vi "svx_DAQ_ConfigureTask.vi"(0 "Task In":T1, 5 "Display State In":T3={"Channel Info Array"=[], "Timing Mode"=enum."Time", "Timing Control 1"=25600.0, "Timing Control 2"=2560.0, "Timing Control 3"=16, "Timing Indicator 1"=0.1, "Reference Visible?"=FALSE, "Reference Type"=enum."<none>", "Tachometer Channel"="", "Tach Pulses Per Rev"=1, "Tach Direction"=enum."CW", "Tach Slope"=enum."Rising", "Tach Threshold"=0.0, "Trigger Channel"="", "Trigger Level"=20.0, "Pretrigger Samples"=1, "Trigger Slope"=enum."Falling", "Trigger Hysteresis"=0.0, "Logging Visible?"=FALSE, "Enable Logging"=FALSE, "Logfile Path"=path "c:/test.tdms"} caption="State" {"Timing Control 2" format="%#_6f"; "Channel Info Array"."Max" min=0.0 format="± %^#_4g"; "Channel Info Array"."Channel Type" items=["Voltage (V)"=0, "Charge (C)"=9, "-"=99, "SPL (Pa)"=3, "Force (lbf)"=6, "Force (N)"=1, "Acceleration (g) - IEPE"=2, "Acceleration (g) - Charge"=12, "Acceleration (g) - 4 wire DC Voltage"=22, "Velocity (in/s)"=7, "Velocity (mm/s)"=8, "Prox Probe (mil)"=4, "Prox Probe (mm)"=5]}, 9 "cluster":T2, 11 "error in":errorcluster) -> (4 "task out":refnum<k21>, 6 "Display State Out":T3={"Channel Info Array"=[], "Timing Mode"=enum."Time", "Timing Control 1"=25600.0, "Timing Control 2"=2560.0, "Timing Control 3"=16, "Timing Indicator 1"=0.1, "Reference Visible?"=FALSE, "Reference Type"=enum."<none>", "Tachometer Channel"="", "Tach Pulses Per Rev"=1, "Tach Direction"=enum."CW", "Tach Slope"=enum."Rising", "Tach Threshold"=0.0, "Trigger Channel"="", "Trigger Level"=20.0, "Pretrigger Samples"=1, "Trigger Slope"=enum."Falling", "Trigger Hysteresis"=0.0, "Logging Visible?"=FALSE, "Enable Logging"=FALSE, "Logfile Path"=path "c:/test.tdms"} caption="State" {"Timing Control 2" format="%#_6f"; "Channel Info Array"."Max" min=0.0 format="± %^#_4g"; "Channel Info Array"."Channel Type" items=["Voltage (V)"=0, "Charge (C)"=9, "-"=99, "SPL (Pa)"=3, "Force (lbf)"=6, "Force (N)"=1, "Acceleration (g) - IEPE"=2, "Acceleration (g) - Charge"=12, "Acceleration (g) - 4 wire DC Voltage"=22, "Velocity (in/s)"=7, "Velocity (mm/s)"=8, "Prox Probe (mil)"=4, "Prox Probe (mm)"=5]}, 10 "cluster":T2, 15 "error out":errorcluster)   [LabVIEW 2017, in "SVX NI-DAQmx AI Configuration XControl.xctl"]
uses:
  <vilib>/addons/Sound and Vibration/svt_DAQmx/Configuration XControl/SVX NI-DAQmx AI Configuration XControl.xctl
  <vilib>/addons/Sound and Vibration/svt_DAQmx/Configuration XControl/SubVIs/svx_DAQ_State.ctl
  <vilib>/addons/Sound and Vibration/svt_DAQmx/Configuration XControl/Controls/svx_DAQ_ChannelInfo.ctl
  <vilib>/addons/Sound and Vibration/svt_DAQmx/Configuration XControl/Controls/svx_DAQ_ChannelType.ctl
  <vilib>/addons/Sound and Vibration/svt_DAQmx/Configuration XControl/Controls/svx_DAQ_Coupling.ctl
  <vilib>/addons/Sound and Vibration/svt_DAQmx/Configuration XControl/Controls/svx_DAQ_Excitation.ctl
  <vilib>/addons/Sound and Vibration/svt_DAQmx/Configuration XControl/Controls/svx_DAQ_TimingType.ctl
  <vilib>/addons/Sound and Vibration/svt_DAQmx/Configuration XControl/Controls/svx_DAQ_ReferenceType.ctl
  <vilib>/addons/Sound and Vibration/svt_DAQmx/Configuration XControl/Controls/svx_DAQ_RotationDirection.ctl
  <vilib>/addons/Sound and Vibration/svt_DAQmx/Configuration XControl/Controls/svx_DAQ_Tach_Slope.ctl
  <vilib>/addons/Sound and Vibration/svt_DAQmx/Configuration XControl/Controls/svx_DAQ_Trigger_Slope.ctl
  <vilib>/addons/Sound and Vibration/svt_DAQmx/Configuration XControl/Controls/svx_DAQ_ControlRefs.ctl
  <vilib>/addons/Sound and Vibration/svt_DAQmx/Configuration XControl/SubVIs/svx_DAQ_Data.ctl
  <resource>/objmgr/daqmx.rc
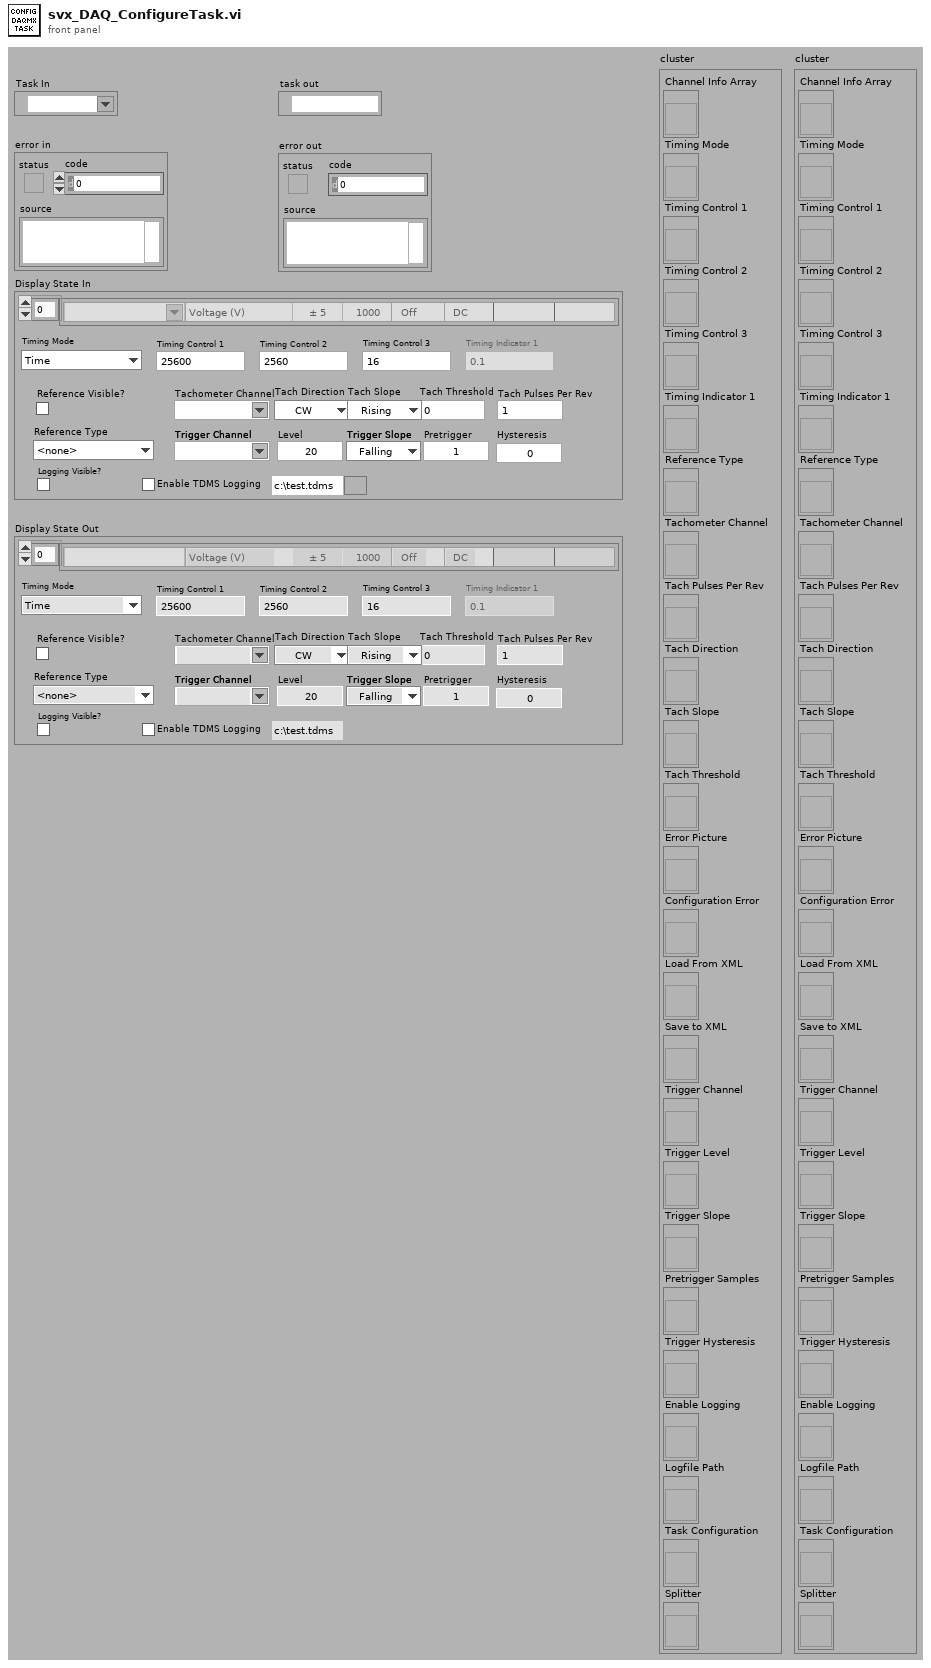
[diagram p1: front panel]
types:
  T1 = typedef "SVX NI-DAQmx AI Configuration XControl.xctl/svx_DAQ_Data.ctl" = refnum<k21>
  T2 = typedef "SVX NI-DAQmx AI Configuration XControl.xctl/svx_DAQ_ControlRefs.ctl" = cluster{"Channel Info Array":refnum<vi>, "Timing Mode":refnum<vi>, "Timing Control 1":refnum<vi>, "Timing Control 2":refnum<vi>, "Timing Control 3":refnum<vi>, "Timing Indicator 1":refnum<vi>, "Reference Type":refnum<vi>, "Tachometer Channel":refnum<vi>, "Tach Pulses Per Rev":refnum<vi>, "Tach Direction":refnum<vi>, "Tach Slope":refnum<vi>, "Tach Threshold":refnum<vi>, "Error Picture":refnum<vi>, "Configuration Error":refnum<vi>, "Load From XML":refnum<vi>, "Save to XML":refnum<vi>, "Trigger Channel":refnum<vi>, "Trigger Level":refnum<vi>, "Trigger Slope":refnum<vi>, "Pretrigger Samples":refnum<vi>, "Trigger Hysteresis":refnum<vi>, "Enable Logging":refnum<vi>, "Logfile Path":refnum<vi>, "Task Configuration":refnum<vi>, "Splitter":refnum<vi>}
  T3 = typedef "SVX NI-DAQmx AI Configuration XControl.xctl/svx_DAQ_State.ctl" = cluster{"Channel Info Array":T4[], "Timing Mode":T8, "Timing Control 1":dbl, "Timing Control 2":dbl, "Timing Control 3":i32, "Timing Indicator 1":dbl, "Reference Visible?":bool, "Reference Type":T9, "Tachometer Channel":string, "Tach Pulses Per Rev":i32, "Tach Direction":T10, "Tach Slope":T11, "Tach Threshold":dbl, "Trigger Channel":string, "Trigger Level":dbl, "Pretrigger Samples":i32, "Trigger Slope":T12, "Trigger Hysteresis":dbl, "Logging Visible?":bool, "Enable Logging":bool, "Logfile Path":path}
  T4 = typedef "SVX NI-DAQmx AI Configuration XControl.xctl/svx_DAQ_ChannelInfo.ctl" = cluster{"Initialized?":bool, "DAQmx Channel":tag, "Channel Type":T5, "Max":dbl, "Sensitivity":dbl, "Excitation":bool, "Coupling":T6, "Location":string, "Orientation":string, "excitation":T7}
  T5 = typedef "SVX NI-DAQmx AI Configuration XControl.xctl/svx_DAQ_ChannelType.ctl" = u16
  T6 = typedef "SVX NI-DAQmx AI Configuration XControl.xctl/svx_DAQ_Coupling.ctl" = enum16{"AC", "DC"}
  T7 = typedef "svx_DAQ_Excitation.ctl" = enum16{"Off", "Min", "Max"}
  T8 = typedef "SVX NI-DAQmx AI Configuration XControl.xctl/svx_DAQ_TimingType.ctl" = enum16{"Time", "Frequency", "Order"}
  T9 = typedef "SVX NI-DAQmx AI Configuration XControl.xctl/svx_DAQ_ReferenceType.ctl" = enum16{"<none>", "Analog Tachometer", "Analog SW Trigger"}
  T10 = typedef "SVX NI-DAQmx AI Configuration XControl.xctl/svx_DAQ_RotationDirection.ctl" = enum16{"CW", "CCW"}
  T11 = typedef "SVX NI-DAQmx AI Configuration XControl.xctl/svx_DAQ_Tach_Slope.ctl" = enum16{"Rising", "Falling"}
  T12 = typedef "SVX NI-DAQmx AI Configuration XControl.xctl/svx_DAQ_Trigger_Slope.ctl" = enum16{"Falling", "Rising"}
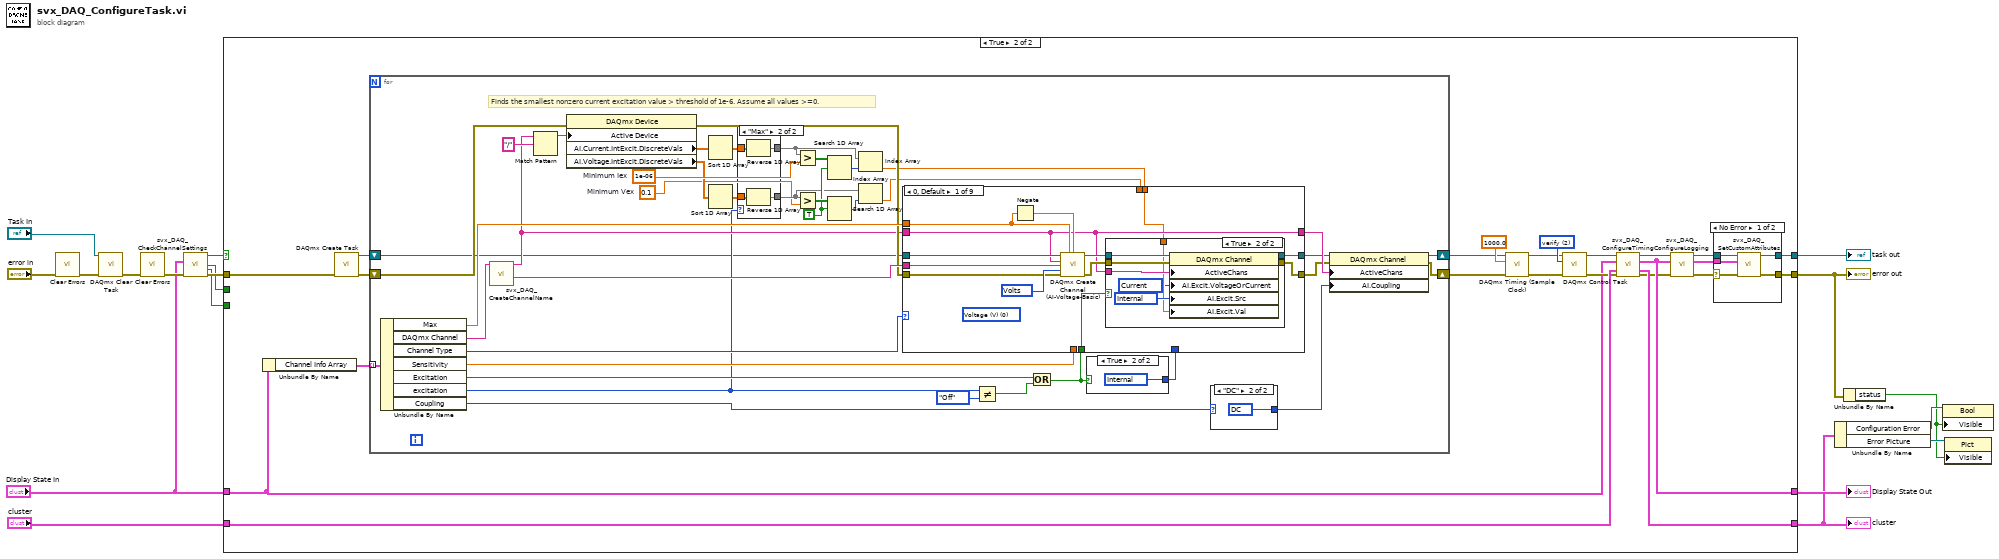
[diagram p0: block diagram]
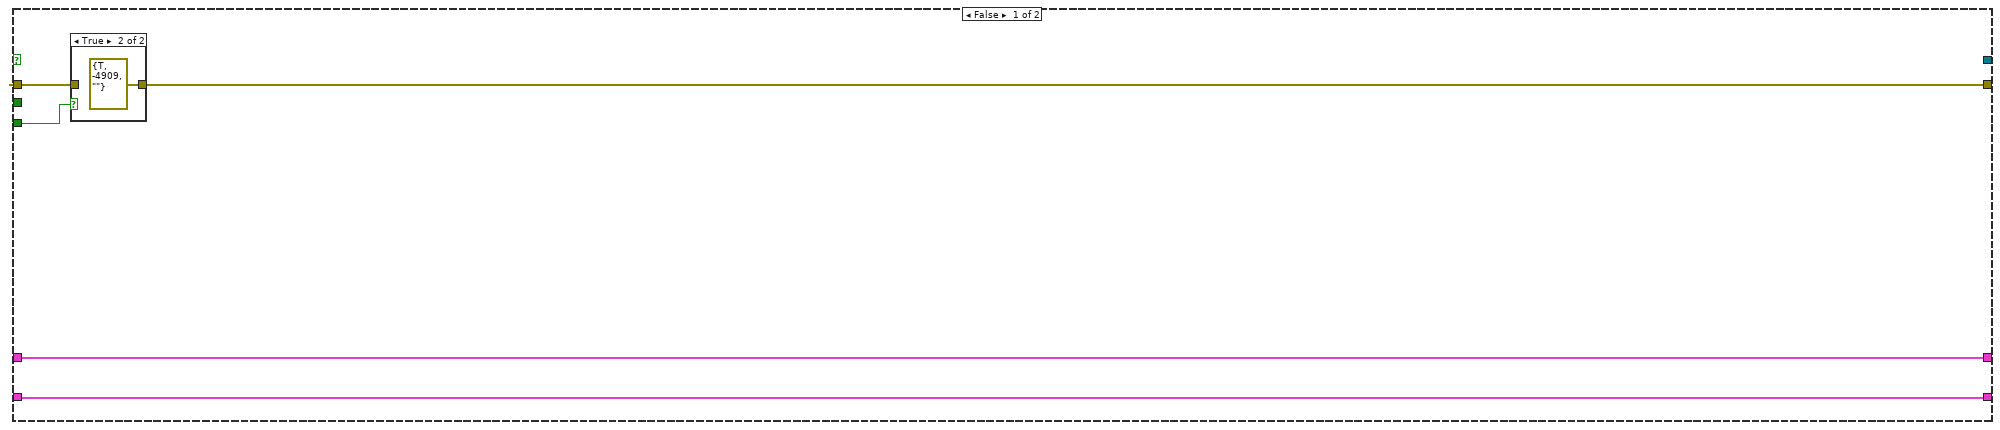
[diagram p2: hidden frame]
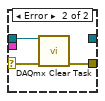
[diagram p5: hidden frame]
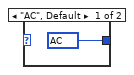
[diagram p7: hidden frame]
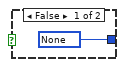
[diagram p8: hidden frame]
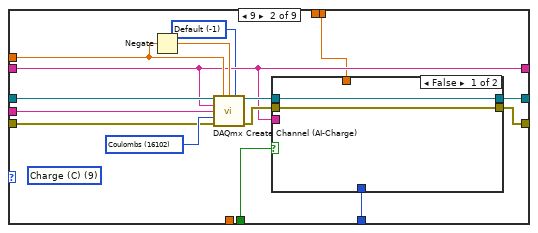
[diagram p10: hidden frame]
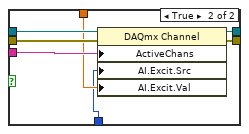
[diagram p11: hidden frame]
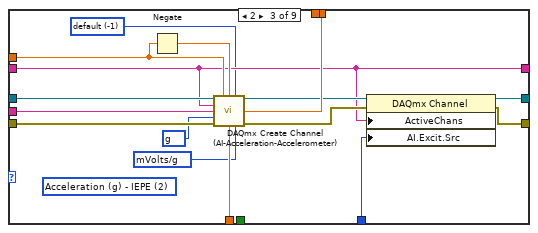
[diagram p12: hidden frame]
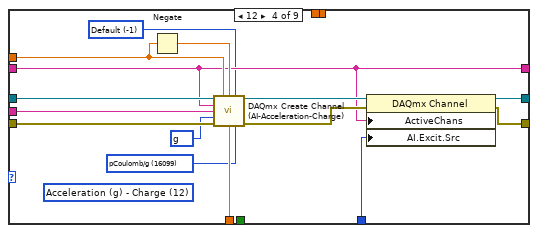
[diagram p13: hidden frame]
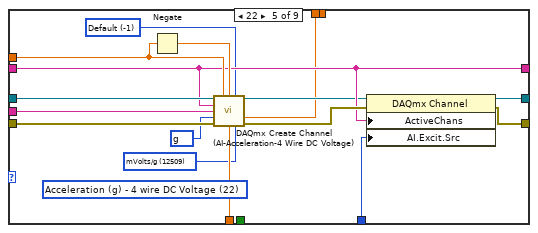
[diagram p14: hidden frame]
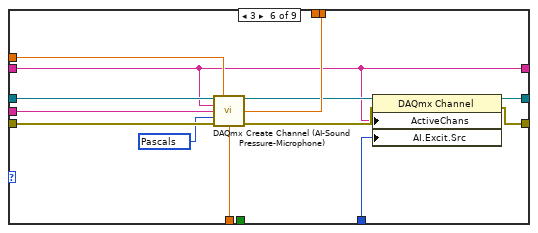
[diagram p15: hidden frame]
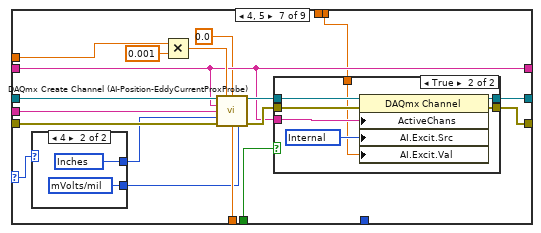
[diagram p16: hidden frame]
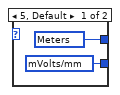
[diagram p17: hidden frame]
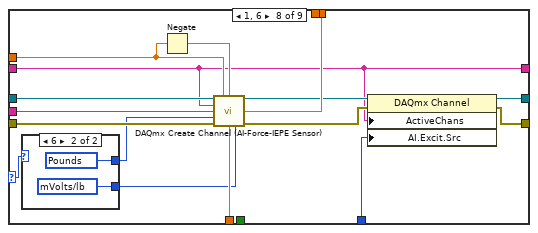
[diagram p19: hidden frame]
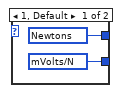
[diagram p20: hidden frame]
diagram:
  n1 = call <vilib>:"Clear Errors.vi"("error in (no error)"="error in") -> ("error out"=w9:errorcluster)  [unwired: 5 in, 1 out]
  n2 = call <vilib>:"DAQmx Clear Task.vi"("task in"="Task In", "error in"=w9) -> ("error out"=w12:errorcluster)  [unwired: 13 in]
  n3 = call <vilib>:"Clear Errors.vi"("error in (no error)"=w12) -> ("error out"=w6:errorcluster)  [unwired: 5 in, 1 out]
  n4 = call <vilib>:"svx_DAQ_CheckChannelSettings.vi"("Display State In"="Display State In", "error in (no error)"=w6) -> ("Configure DAQ Settings?"=w11:bool, "Tach Channel Invalid"=w3:bool, "Trigger Channel Invalid"=w2:bool, "error out"=w5:errorcluster)  [unwired: 9 in, 1 out]
  n5 = case shown="True" w11 {
    tunnel: [_ w48] -> w18
    tunnel: [w19 w49] -> w14
    tunnel: [w24 w38] -> w15
    tunnel: w5 -> [w22 w50]
    tunnel: "cluster" -> [w25 w47]
    tunnel: [w25 w46] -> w7
    tunnel: "Display State In" -> [w24 w41]
    tunnel: w3 -> [w21 _]
    tunnel: w2 -> [w20 _]
    frame False {
      n6 = case shown="True" w21 {
        tunnel: [w28 errorcluster {"status"=TRUE, "code"=-4908, "source"=""} ("error out")] -> w23
        tunnel: w22 -> [w28 _]
        frame False {
        }
        frame True {
        }
      }
      n7 = case shown="True" w20 {
        tunnel: w23 -> [w26 _]
        tunnel: [w26 errorcluster {"status"=TRUE, "code"=-4909, "source"=""} ("error out")] -> w19
        frame False {
        }
        frame True {
        }
      }
    }
    frame True {
      w44 = 2 items=["verify"=2, "reserve"=4, "commit"=3, "unreserve"=5, "abort"=6] ("action")
      n8 = Unbundle By Name(w41) -> ("Channel Info Array"=w42:T4[])
      n9 = call <vilib>:"DAQmx Create Task.vi"("error in"=w50) -> ("task out"=w52:refnum<k21>, "error out"=w51:errorcluster)  [unwired: 13 in]
      n10 = for {
        tunnel: w42 -> [w98] mode=indexing
        shift-right: [w89] -> w32
        shift-left: w51 -> [w84]
        shift-right: [w90] -> w33
        shift-left: w52 -> [w61]
        w62 = 0.1  # Minimum Vex
        w69 = TRUE ("element")
        w80 = 1e-06  # Minimum Iex
        # "Finds the smallest nonzero current excitation value > threshold of 1e-6. Assume all values >=0."
        n11 = Unbundle By Name(w98) -> ("Max"=w96:dbl, "DAQmx Channel"=w88:tag, "Channel Type"=w100:T5, "Sensitivity"=w99:dbl, "Excitation"=w74:bool, "excitation"=w63:T7, "Coupling"=w97:T6)
        n12 = call <vilib>:"svx_DAQ_CreateChannelName.vi"("DAQmx Channel In"=w88) -> ("Channel Name"=w87:string, "DAQmx Channel Out"=w77:tag)  [unwired: 9 in]
        n13 = Match Pattern(string=w77, regular expression="/") -> (before substring=w85:string)  [unwired: 1 in, 3 out]
        n14 = property class="DAQmx Device"(error in=w84, "Active Device"=w85) -> (error out=w83:errorcluster, "AI.Current.IntExcit.DiscreteVals"=w82:dbl[], "AI.Voltage.IntExcit.DiscreteVals"=w70:dbl[])  [unwired: 1 in, 1 out]
        n15 = Sort 1D Array(array=w82) -> (sorted array=w66:dbl[])
        n16 = Sort 1D Array(array=w70) -> (sorted array=w64:dbl[])
        n17 = case shown="\"Max\"" w63 {
          tunnel: [w102 w104] -> w67
          tunnel: w66 -> [w102 w106]
          tunnel: [w101 w103] -> w65
          tunnel: w64 -> [w101 w105]
          frame "Off", "Min", Default {
          }
          frame "Max" {
            n18 = Reverse 1D Array(array=w106) -> (reversed array=w104:dbl[])
            n19 = Reverse 1D Array(array=w105) -> (reversed array=w103:dbl[])
          }
        }
        n20 = Greater?(x=w67, y=w80) -> (0:w79:bool[])
        n21 = Greater?(x=w65, y=w62) -> (0:w71:bool[])
        n22 = Search 1D Array(1D array=w79, element=w69) -> (index of element=w78:i32)  [unwired: 1 in]
        n23 = Search 1D Array(1D array=w71, element=w69) -> (index of element=w72:i32)  [unwired: 1 in]
        n24 = Index Array(array=w67, index=w78) -> (element=w81:dbl)
        n25 = Index Array(array=w65, index=w72) -> (element=w68:dbl)
        n26 = Not Equal?(x=w63, y=svx_DAQ_Excitation."Off") -> (x != y?=w75:bool)
        n27 = Or(x=w74, y=w75) -> (x .or. y?=w73:bool)
        n28 = case shown="True" w73 {
          tunnel: [w109 w110] -> w93
          frame False {
            w109 = 10230 items=["Internal"=10200, "External"=10167, "None"=10230] ("AI.Excit.Src")
          }
          frame True {
            w110 = 10200 items=["Internal"=10200, "External"=10167, "None"=10230] ("AI.Excit.Src")
          }
        }
        n29 = case shown="0, Default" w100 {
          selector: w100 -> [_ _ _ _ _ _ w221 w251 w282]
          tunnel: w61 -> [w123 w148 w173 w188 w204 w217 w235 w264 w277]
          tunnel: w77 -> [w113 w138 w163 w180 w197 w208 w226 w254 w276]
          tunnel: w96 -> [w121 w146 w172 w187 w203 w216 w231 w261 w281]
          tunnel: w99 -> [_ _ w168 w183 w199 w214 w233 w262 w273]
          tunnel: w83 -> [w119 w144 w170 w185 w201 w215 w234 w263 w272]
          tunnel: [w116 w141 w160 w177 w194 w211 w225 w258 w285] -> w92
          tunnel: [w115 w140 w161 w178 w195 w206 w224 w257 w284] -> w91
          tunnel: [w113 w138 w163 w180 w197 w208 w226 w254 w276] -> w94
          tunnel: w73 -> [w114 w139 _ _ _ _ w229 _ _]
          tunnel: w81 -> [w111 w136 w166 _ _ w212 w218 w259 w278]
          tunnel: w93 -> [_ w134 w162 w179 w196 w207 _ w253 w283]
          tunnel: w87 -> [w112 w137 w159 w176 w193 w205 w222 w252 w271]
          tunnel: w68 -> [_ _ _ _ w189 _ _ _ _]
          frame 0, Default {
            (unwired) T5 0 items=["Voltage (V)"=0, "Charge (C)"=9, "-"=99, "SPL (Pa)"=3, "Force (lbf)"=6, "Force (N)"=1, "Acceleration (g) - IEPE"=2, "Acceleration (g) - Charge"=12, "Acceleration (g) - 4 wire DC Voltage"=22, "Velocity (in/s)"=7, "Velocity (mm/s)"=8, "Prox Probe (mil)"=4, "Prox Probe (mm)"=5] ("Channel Type")
            w122 = 10348 items=["Volts"=10348, "From Custom Scale"=10065] ("units")
            n30 = Negate(x=w121) -> (-x=w120:dbl)
            n31 = call <vilib>:"DAQmx Create Channel (AI-Voltage-Basic).vi"("task in"=w123, "maximum value"=w121, "minimum value"=w120, "physical channels"=w113, "name to assign"=w112, "units"=w122, "error in"=w119) -> ("task out"=w118:refnum<k21>, "error out"=w117:errorcluster)  [unwired: 7 in]
            n32 = case shown="True" w114 {
              tunnel: w118 -> [w125 w133]
              tunnel: w117 -> [w124 w132]
              tunnel: w113 -> [_ w131]
              tunnel: [w125 w130] -> w116
              tunnel: [w124 w129] -> w115
              tunnel: w111 -> [_ w127]
              frame False {
              }
              frame True {
                w126 = 10134 items=["Voltage"=10322, "Current"=10134] ("AI.Excit.VoltageOrCurrent")
                w128 = 10200 items=["Internal"=10200, "External"=10167, "None"=10230] ("AI.Excit.Src")
                n33 = property class="DAQmx Channel"(reference=w133, error in=w132, "ActiveChans"=w131, "AI.Excit.VoltageOrCurrent"=w126, "AI.Excit.Src"=w128, "AI.Excit.Val"=w127) -> (reference out=w130:refnum<k21>, error out=w129:errorcluster)
              }
            }
          }
          frame 9 {
            (unwired) T5 9 items=["Voltage (V)"=0, "Charge (C)"=9, "-"=99, "SPL (Pa)"=3, "Force (lbf)"=6, "Force (N)"=1, "Acceleration (g) - IEPE"=2, "Acceleration (g) - Charge"=12, "Acceleration (g) - 4 wire DC Voltage"=22, "Velocity (in/s)"=7, "Velocity (mm/s)"=8, "Prox Probe (mil)"=4, "Prox Probe (mm)"=5] ("Channel Type")
            w135 = -1 items=["Default"=-1, "RSE"=10083, "NRSE"=10078, "Differential"=10106, "Pseudodifferential"=12529] ("input terminal configuration")
            w147 = 16102 items=["Coulombs"=16102, "pCoulombs"=16103, "From Custom Scale"=10065] ("units")
            n34 = Negate(x=w146) -> (-x=w145:dbl)
            n35 = call <vilib>:"DAQmx Create Channel (AI-Charge).vi"("task in"=w148, "maximum value"=w146, "minimum value"=w145, "input terminal configuration"=w135, "physical channels"=w138, "name to assign"=w137, "units"=w147, "error in"=w144) -> ("task out"=w143:refnum<k21>, "error out"=w142:errorcluster)  [unwired: 6 in]
            n36 = case shown="False" w139 {
              tunnel: w143 -> [w150 w157]
              tunnel: w142 -> [w149 w156]
              tunnel: w138 -> [_ w155]
              tunnel: [w150 w154] -> w141
              tunnel: [w149 w153] -> w140
              tunnel: w136 -> [_ w152]
              tunnel: w134 -> [_ w151]
              frame False {
              }
              frame True {
                n37 = property class="DAQmx Channel"(reference=w157, error in=w156, "ActiveChans"=w155, "AI.Excit.Src"=w151, "AI.Excit.Val"=w152) -> (reference out=w154:refnum<k21>, error out=w153:errorcluster)
              }
            }
          }
          frame 2 {
            w158 = -1 items=["default"=-1, "RSE"=10083, "NRSE"=10078, "Differential"=10106, "Pseudodifferential"=12529] ("input terminal configuration")
            (unwired) T5 2 items=["Voltage (V)"=0, "Charge (C)"=9, "-"=99, "SPL (Pa)"=3, "Force (lbf)"=6, "Force (N)"=1, "Acceleration (g) - IEPE"=2, "Acceleration (g) - Charge"=12, "Acceleration (g) - 4 wire DC Voltage"=22, "Velocity (in/s)"=7, "Velocity (mm/s)"=8, "Prox Probe (mil)"=4, "Prox Probe (mm)"=5] ("Channel Type")
            w167 = 12509 items=["mVolts/g"=12509, "Volts/g"=12510] ("sensitivity units")
            w169 = 10186 items=["g"=10186, "m/s^2"=12470, "From Custom Scale"=10065] ("units")
            n38 = Negate(x=w172) -> (-x=w171:dbl)
            n39 = call <vilib>:"DAQmx Create Channel (AI-Acceleration-Accelerometer).vi"("task in"=w173, "maximum value"=w172, "minimum value"=w171, "input terminal configuration"=w158, "physical channels"=w163, "name to assign"=w159, "current excitation value"=w166, "units"=w169, "error in"=w170, "sensitivity"=w168, "sensitivity units"=w167) -> ("task out"=w165:refnum<k21>, "error out"=w164:errorcluster)  [unwired: 3 in]
            n40 = property class="DAQmx Channel"(reference=w165, error in=w164, "ActiveChans"=w163, "AI.Excit.Src"=w162) -> (reference out=w160:refnum<k21>, error out=w161:errorcluster)
          }
          frame 12 {
            w174 = -1 items=["Default"=-1, "RSE"=10083, "NRSE"=10078, "Differential"=10106, "Pseudodifferential"=12529] ("input terminal configuration")
            w175 = 16099 items=["pCoulomb/g"=16099, "pCoulomb/(m/s^2)"=16100, "pCoulomb/(in/s^2)"=16101] ("sensitivity units")
            (unwired) T5 12 items=["Voltage (V)"=0, "Charge (C)"=9, "-"=99, "SPL (Pa)"=3, "Force (lbf)"=6, "Force (N)"=1, "Acceleration (g) - IEPE"=2, "Acceleration (g) - Charge"=12, "Acceleration (g) - 4 wire DC Voltage"=22, "Velocity (in/s)"=7, "Velocity (mm/s)"=8, "Prox Probe (mil)"=4, "Prox Probe (mm)"=5] ("Channel Type")
            w184 = 10186 items=["g"=10186, "m/s^2"=12470, "From Custom Scale"=10065] ("units")
            n41 = Negate(x=w187) -> (-x=w186:dbl)
            n42 = call <vilib>:"DAQmx Create Channel (AI-Acceleration-Charge).vi"("task in"=w188, "maximum value"=w187, "minimum value"=w186, "input terminal configuration"=w174, "physical channels"=w180, "name to assign"=w176, "units"=w184, "error in"=w185, "sensitivity"=w183, "sensitivity units"=w175) -> ("task out"=w182:refnum<k21>, "error out"=w181:errorcluster)  [unwired: 4 in]
            n43 = property class="DAQmx Channel"(reference=w182, error in=w181, "ActiveChans"=w180, "AI.Excit.Src"=w179) -> (reference out=w177:refnum<k21>, error out=w178:errorcluster)
          }
          frame 22 {
            w190 = -1 items=["Default"=-1, "RSE"=10083, "NRSE"=10078, "Differential"=10106, "Pseudodifferential"=12529] ("input terminal configuration")
            w192 = 12509 items=["mVolts/g"=12509, "Volts/g"=12510] ("sensitivity units")
            (unwired) T5 22 items=["Voltage (V)"=0, "Charge (C)"=9, "-"=99, "SPL (Pa)"=3, "Force (lbf)"=6, "Force (N)"=1, "Acceleration (g) - IEPE"=2, "Acceleration (g) - Charge"=12, "Acceleration (g) - 4 wire DC Voltage"=22, "Velocity (in/s)"=7, "Velocity (mm/s)"=8, "Prox Probe (mil)"=4, "Prox Probe (mm)"=5] ("Channel Type")
            w200 = 10186 items=["g"=10186, "m/s^2"=12470, "From Custom Scale"=10065] ("units")
            n44 = Negate(x=w203) -> (-x=w202:dbl)
            n45 = call <vilib>:"DAQmx Create Channel (AI-Acceleration-4 Wire DC Voltage).vi"("task in"=w204, "maximum value"=w203, "minimum value"=w202, "input terminal configuration"=w190, "physical channels"=w197, "name to assign"=w193, "units"=w200, "voltage excitation value"=w189, "error in"=w201, "sensitivity"=w199, "sensitivity units"=w192) -> ("task out"=w191:refnum<k21>, "error out"=w198:errorcluster)  [unwired: 3 in]
            n46 = property class="DAQmx Channel"(reference=w191, error in=w198, "ActiveChans"=w197, "AI.Excit.Src"=w196) -> (reference out=w194:refnum<k21>, error out=w195:errorcluster)
          }
          frame 3 {
            w213 = 10081 items=["Pascals"=10081, "From Custom Scale"=10065] ("units")
            n47 = call <vilib>:"DAQmx Create Channel (AI-Sound Pressure-Microphone).vi"("task in"=w217, "maximum sound pressure level"=w216, "physical channels"=w208, "name to assign"=w205, "current excitation value"=w212, "units"=w213, "error in"=w215, "microphone sensitivity"=w214) -> ("task out"=w210:refnum<k21>, "error out"=w209:errorcluster)  [unwired: 6 in]
            n48 = property class="DAQmx Channel"(reference=w210, error in=w209, "ActiveChans"=w208, "AI.Excit.Src"=w207) -> (reference out=w211:refnum<k21>, error out=w206:errorcluster)
          }
          frame 4, 5 {
            n49 = case shown="4" w221 {
              tunnel: [w237 w239] -> w220
              tunnel: [w236 w238] -> w219
              frame 5, Default {
                w236 = 14838 items=["mVolts/mil"=14836, "Volts/mil"=14837, "mVolts/mm"=14838, "Volts/mm"=14839, "mVolts/micron"=14840] ("sensitivity units")
                w237 = 10219 items=["Meters"=10219, "Inches"=10379, "From Custom Scale"=10065] ("units")
              }
              frame 4 {
                w238 = 14836 items=["mVolts/mil"=14836, "Volts/mil"=14837, "mVolts/mm"=14838, "Volts/mm"=14839, "mVolts/micron"=14840] ("sensitivity units")
                w239 = 10379 items=["Meters"=10219, "Inches"=10379, "From Custom Scale"=10065] ("units")
              }
            }
            n50 = Multiply(x=w231, y=0.001) -> (x*y=w230:dbl)
            n51 = call <vilib>:"DAQmx Create Channel (AI-Position-EddyCurrentProxProbe).vi"("task in"=w235, "maximum value"=w230, "minimum value"=0.0, "physical channels"=w226, "name to assign"=w222, "units"=w220, "error in"=w234, "sensitivity"=w233, "sensitivity units"=w219) -> ("task out"=w227:refnum<k21>, "error out"=w228:errorcluster)  [unwired: 5 in]
            n52 = case shown="True" w229 {
              tunnel: w227 -> [w241 w248]
              tunnel: w228 -> [w240 w247]
              tunnel: w226 -> [_ w246]
              tunnel: [w241 w245] -> w225
              tunnel: [w240 w244] -> w224
              tunnel: w218 -> [_ w242]
              frame False {
              }
              frame True {
                w243 = 10200 items=["Internal"=10200, "External"=10167, "None"=10230] ("AI.Excit.Src")
                n53 = property class="DAQmx Channel"(reference=w248, error in=w247, "ActiveChans"=w246, "AI.Excit.Src"=w243, "AI.Excit.Val"=w242) -> (reference out=w245:refnum<k21>, error out=w244:errorcluster)
              }
            }
          }
          frame 1, 6 {
            n54 = case shown="6" w251 {
              tunnel: [w266 w268] -> w250
              tunnel: [w265 w267] -> w249
              frame 1, Default {
                w265 = 15891 items=["mVolts/N"=15891, "mVolts/lb"=15892] ("sensitivity units")
                w266 = 15875 items=["Newtons"=15875, "Pounds"=15876, "kgf"=15877, "From Custom Scale"=10065] ("units")
              }
              frame 6 {
                w267 = 15892 items=["mVolts/N"=15891, "mVolts/lb"=15892] ("sensitivity units")
                w268 = 15876 items=["Newtons"=15875, "Pounds"=15876, "kgf"=15877, "From Custom Scale"=10065] ("units")
              }
            }
            n55 = Negate(x=w261) -> (-x=w260:dbl)
            n56 = call <vilib>:"DAQmx Create Channel (AI-Force-IEPE Sensor).vi"("task in"=w264, "maximum value"=w261, "minimum value"=w260, "physical channels"=w254, "name to assign"=w252, "current excitation value"=w259, "units"=w250, "error in"=w263, "sensitivity"=w262, "sensitivity units"=w249) -> ("task out"=w256:refnum<k21>, "error out"=w255:errorcluster)  [unwired: 4 in]
            n57 = property class="DAQmx Channel"(reference=w256, error in=w255, "ActiveChans"=w254, "AI.Excit.Src"=w253) -> (reference out=w258:refnum<k21>, error out=w257:errorcluster)
          }
          frame 7, 8 {
            n58 = case shown="8" w282 {
              tunnel: [w288 w293] -> w275
              tunnel: [w287 w292] -> w274
              tunnel: w281 -> [w286 w290]
              tunnel: [w286 w289] -> w280
              frame 7, Default {
                w287 = 15964 items=["mVolts/mm/s"=15963, "mVolts/in/s"=15964] ("sensitivity units")
                w288 = 15960 items=["m/s"=15959, "in/s"=15960, "From Custom Scale"=10065] ("units")
              }
              frame 8 {
                w292 = 15963 items=["mVolts/mm/s"=15963, "mVolts/in/s"=15964] ("sensitivity units")
                w293 = 15959 items=["m/s"=15959, "in/s"=15960, "From Custom Scale"=10065] ("units")
                n59 = Multiply(x=w290, y=0.001) -> (x*y=w289:dbl)
              }
            }
            n60 = Negate(x=w280) -> (-x=w279:dbl)
            n61 = call <vilib>:"DAQmx Create Channel (AI-Velocity-IEPE Sensor).vi"("task in"=w277, "maximum value"=w280, "minimum value"=w279, "physical channels"=w276, "name to assign"=w271, "current excitation value"=w278, "units"=w275, "error in"=w272, "sensitivity"=w273, "sensitivity units"=w274) -> ("task out"=w270:refnum<k21>, "error out"=w269:errorcluster)  [unwired: 4 in]
            n62 = property class="DAQmx Channel"(reference=w270, error in=w269, "ActiveChans"=w276, "AI.Excit.Src"=w283) -> (reference out=w285:refnum<k21>, error out=w284:errorcluster)
          }
        }
        n63 = case shown="\"DC\"" w97 {
          tunnel: [w107 w108] -> w95
          frame "AC", Default {
            w107 = 10045 items=["AC"=10045, "DC"=10050, "GND"=10066] ("AI.Coupling")
          }
          frame "DC" {
            w108 = 10050 items=["AC"=10045, "DC"=10050, "GND"=10066] ("AI.Coupling")
          }
        }
        n64 = property class="DAQmx Channel"(reference=w92, error in=w91, "ActiveChans"=w94, "AI.Coupling"=w95) -> (reference out=w90:refnum<k21>, error out=w89:errorcluster)
      }
      n65 = call <vilib>:"DAQmx Timing (Sample Clock).vi"("task/channels in"=w33, "rate"=1000.0, "error in"=w32) -> ("task out"=w31:refnum<k21>, "error out"=w30:errorcluster)  [unwired: 11 in]
      n66 = call <vilib>:"DAQmx Control Task.vi"("task/channels in"=w31, "action"=w44, "error in"=w30) -> ("task out"=w43:refnum<k21>, "error out"=w45:errorcluster)  [unwired: 11 in]
      n67 = call <vilib>:"svx_DAQ_ConfigureTiming.vi"("Task In"=w43, "Display State In"=w41, "cluster"=w47, "Error In (no error)"=w45) -> ("task out"=w40:refnum<k21>, "Display State Out"=w38:T3, "cluster"=w46:T2, "error out"=w36:errorcluster)  [unwired: 8 in]
      n68 = call <vilib>:"svx_DAQ_ConfigureLogging.vi"("Task In"=w40, "Display State In"=w38, "Error In (no error)"=w36) -> ("task out"=w39:refnum<k21>, "Display State Out"=w37:T3, "error out"=w35:errorcluster)  [unwired: 10 in]
      n69 = case shown="No Error" w35 {
        selector: w35 -> [w54 w59]
        tunnel: [w57 _] -> w48
        tunnel: w37 -> [w53 _]
        tunnel: w39 -> [w56 w60]
        tunnel: [w55 w58] -> w49
        frame No Error {
          n70 = call <vilib>:"svx_DAQ_SetCustomAttributes.vi"("task in"=w56, "Display State In"=w53, "error in (no error)"=w54) -> ("task out"=w57:refnum<k21>, "error out"=w55:errorcluster)  [unwired: 11 in]
        }
        frame Error {
          n71 = call <vilib>:"DAQmx Clear Task.vi"("task in"=w60, "error in"=w59) -> ("error out"=w58:errorcluster)  [unwired: 13 in]
        }
      }
    }
  }
  "task out" <- w18
  "error out" <- w14
  "Display State Out" <- w15
  "cluster" <- w7
  n72 = Unbundle By Name(w7) -> ("Configuration Error"=w16:refnum<vi>, "Error Picture"=w17:refnum<vi>)
  n73 = Unbundle By Name(w14) -> ("status"=w13:bool)
  n74 = property class="Bool"(reference=w16, "Visible"=w13) -> ()  [unwired: 1 in, 2 out]
  n75 = property class="Pict"(reference=w17, "Visible"=w13) -> ()  [unwired: 1 in, 2 out]
